vi "NanoBright Acquisition self-aligning source code.vi"(1 "Acquisition\nTime (s)":u32=10, 2 "Number \nof files":i32=5 min=1 max=99 step=1, 3 "Acquisition Rate (Hz)":dbl=1000.0 caption="Acquisition\nRate (Hz)") -> ()   [LabVIEW 2014]
uses:
  C:/Program Files (x86)/National Instruments/LabVIEW 2014/vi.lib/ULx/ULx_LV.dll
  Program Files (x86)/National Instruments/LabVIEW 2014/vi.lib/ULx/ULx_LV.dll
  <vilib>/Utility/error.llb/DialogType.ctl
  <vilib>/Analysis/baseanly.llb/Mean (DBL).vi
  <vilib>/ULx/Create Channel.llb/ULx Create Channel (CI-Count Edges).vi
  <vilib>/ULx/Timing.llb/ULx Timing (Sample Clock).vi
  <vilib>/ULx/Read.llb/ULx Read (Counter 1D U32 1Chan NSamp).vi
  <vilib>/Utility/file.llb/Read From Spreadsheet File (DBL).vi
  <vilib>/Analysis/NI_AALBase.lvlib
panel:
  in  "Instrument Key":string="COM3"
  in  "Align after # of loops":dbl=2.0
  in  "Period of measurement (min)":u32=1
  out "concatenated string":string="20_30"
  out "Buffer":dbl=100.0
  out "Samples/loop":i32=10
  in  "File Prefix":string="testa"
  out "Current File":i32=1 format="%1.0f"
  out "Channel 1":dbl=nan format="%#_3g"
  out "Signal":u32[][](graph)
  in  "Clock Source":i32(ring) items=["OnboardClock", "ExternalClock", "NoClock"]
  in  "Count Direction":i32(ring) items=["CountUp", "CountDown"]
  in  "Edge":i32(ring) items=["Rising", "Falling"]
  in  "Counter(s)":refnum<k21>="Dev0/Ci0"
  in  "Initial Count":u32
  in  "stop":bool
  # "Signal Averages"
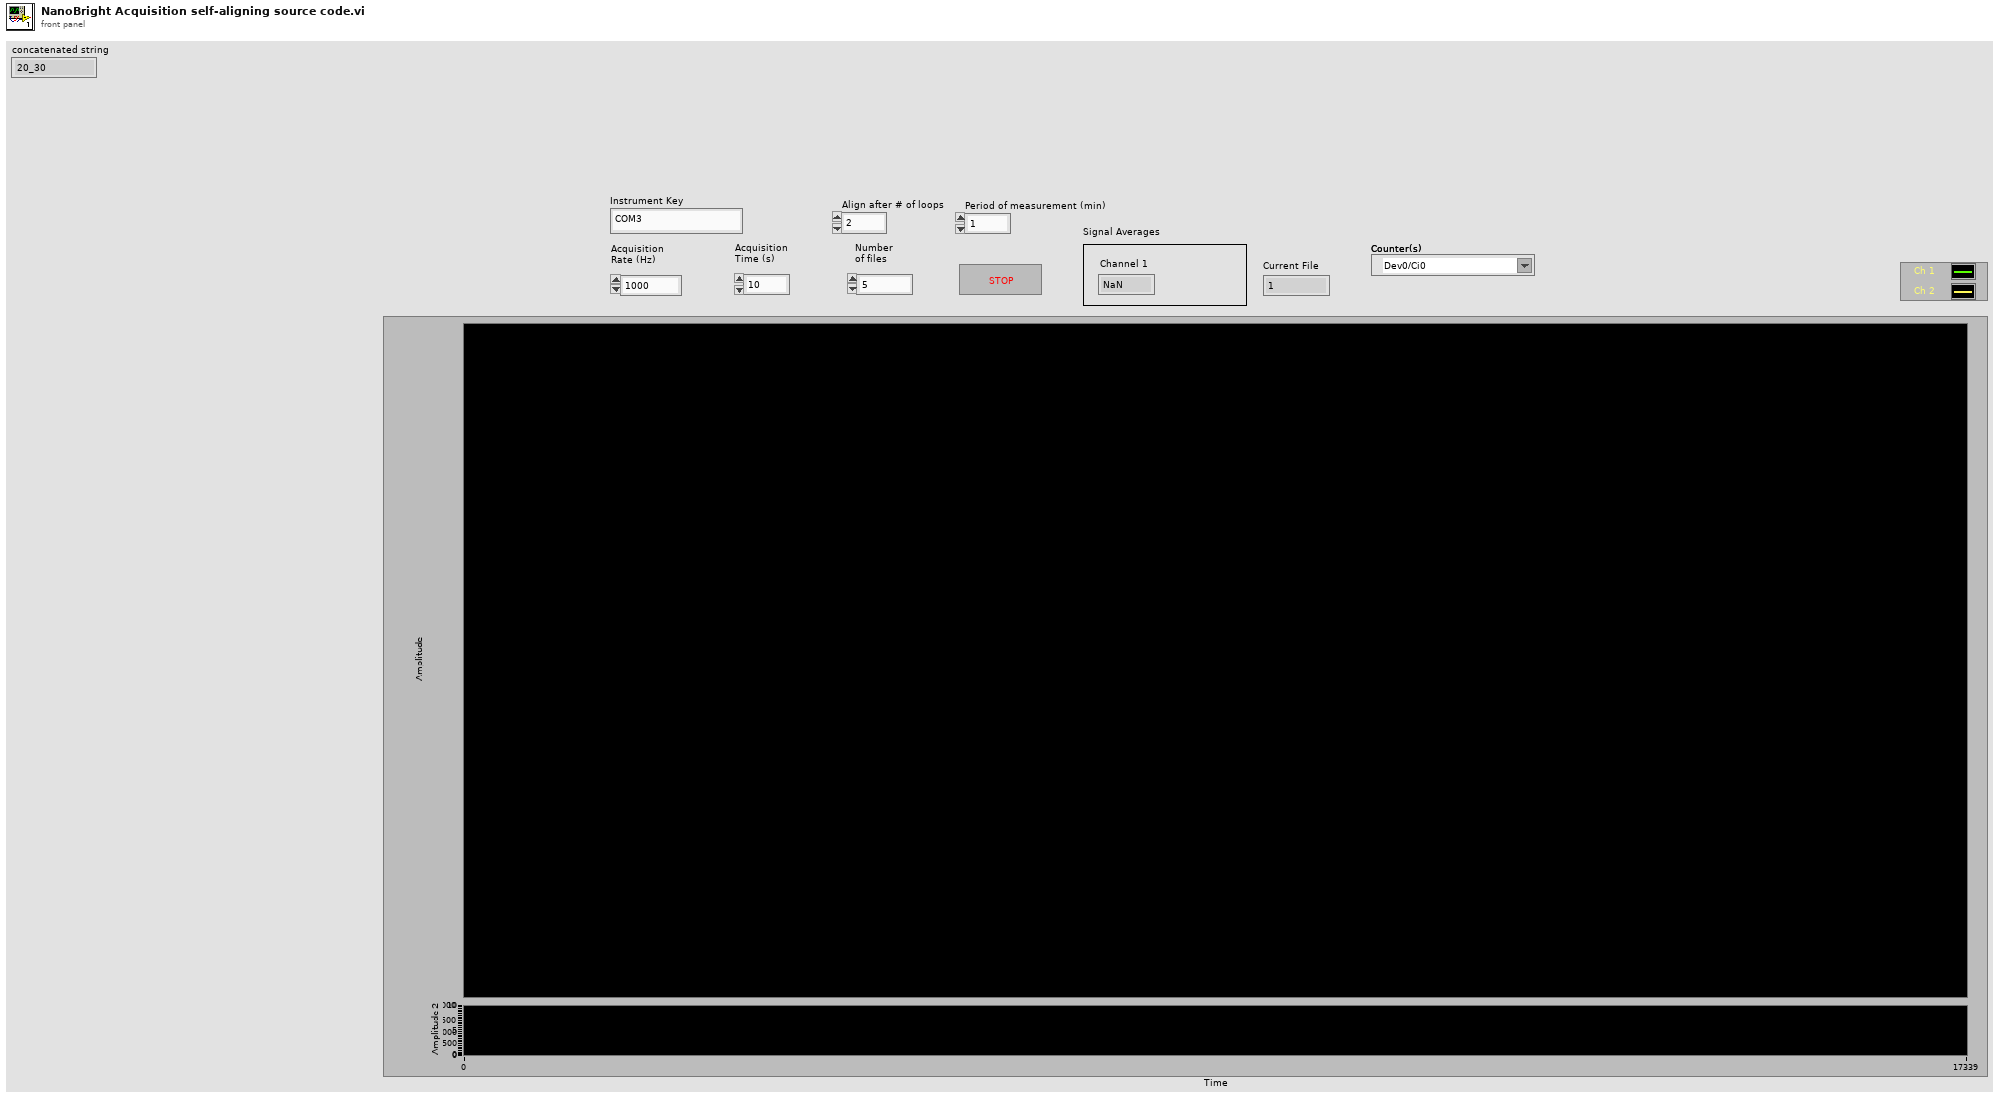
[diagram p1: front panel]
types:
  T1 = enum16{"open", "replace", "create", "open or create", "replace or create", "replace or create with confirmation"}
  T2 = typedef "DialogType.ctl" = u16
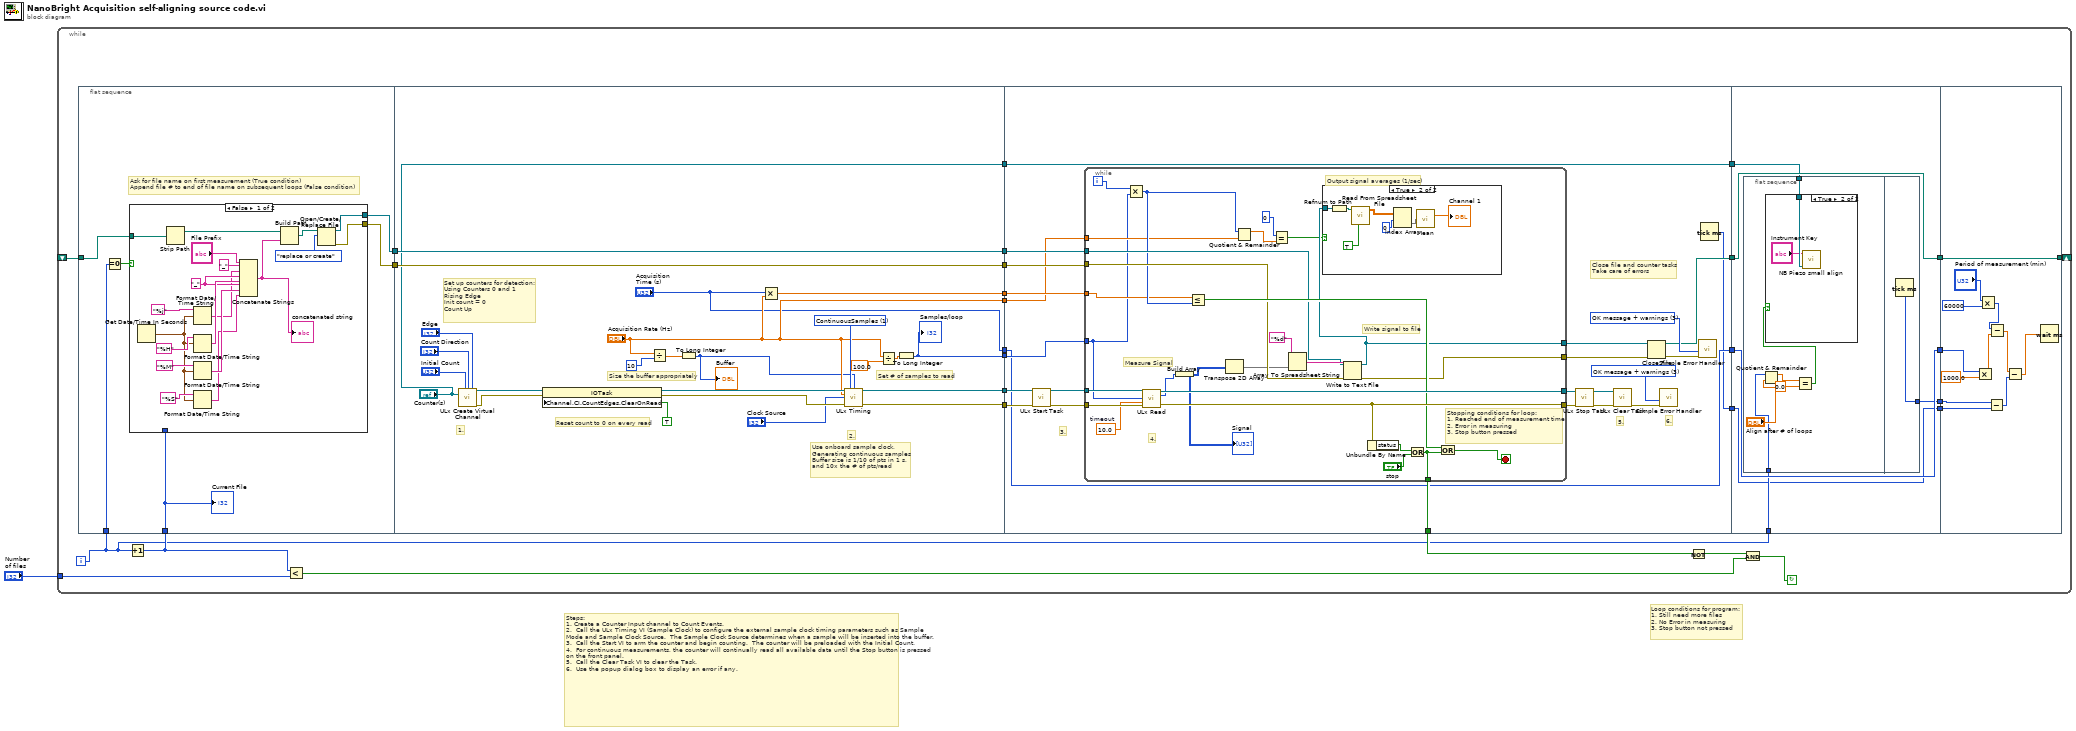
[diagram p0: block diagram]
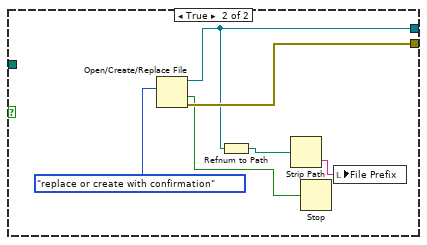
[diagram p2: hidden frame]
diagram:
  # "Loop conditions for program:\n1. Still need more files\n2. No Error in measuring\n3. Stop button not pressed"
  # "Steps: \n1. Create a Counter Input channel to Count Events.\n2.  Call the ULx Timing VI (Sample Clock) to configure the external sample clock timing parameters such as Sample Mode and Sample Clock Source.  The Sample Clock Source determines when a sample will be inserted into the buffer.\n3.  Call the Start VI to arm the counter and begin counting.  The counter will be preloaded with the Initial Count.\n4.  For continuous measurements, the counter will continually read all available data until the Stop button is pressed on the front panel.\n5.  Call the Clear Task VI to clear the Task.\n6.  Use the popup dialog box to display an error if any."
  n1 = while {
    tunnel: "Number \nof files" -> [w21]
    shift-right: [w16] -> _
    shift-left: _ -> [w17]
    i -> [w7]
    stop <- w20 continue-if-true
    n2 = flat-sequence {
      tunnel: [w32] -> w29
      tunnel: [w31] -> w28
      tunnel: w22 -> [w33]
      tunnel: w17 -> [w30]
      tunnel: w7 -> [w34]
      tunnel: [w84] -> w27
      tunnel: [w83] -> w26
      tunnel: [w74] -> w25
      tunnel: [w72] -> w24
      tunnel: [w73] -> w23
      tunnel: w29 -> [w84]
      tunnel: w28 -> [w83]
      tunnel: ["Acquisition Rate (Hz)"] -> w14
      tunnel: [w64] -> w13
      tunnel: ["Acquisition\nTime (s)"] -> w12
      tunnel: ["Counter(s)"] -> w5
      tunnel: w27 -> [w104]
      tunnel: w26 -> [w98]
      tunnel: w25 -> [w94]
      tunnel: w24 -> [w93]
      tunnel: w23 -> [w92]
      tunnel: [w91] -> w19
      tunnel: w14 -> [w89]
      tunnel: w13 -> [w88]
      tunnel: [w90] -> w11
      tunnel: w12 -> [w87]
      tunnel: [w87] -> w9
      tunnel: [w86] -> w6
      tunnel: w5 -> [w86]
      tunnel: [w85] -> w3
      tunnel: w11 -> [w148]
      tunnel: [w148] -> w10
      tunnel: w9 -> [w147]
      tunnel: [w147] -> w8
      tunnel: w7 -> [w146]
      tunnel: w6 -> [w145]
      tunnel: [w144] -> w4
      tunnel: w3 -> [w144]
      tunnel: [w143] -> w2
      tunnel: [w169] -> w16
      tunnel: w10 -> [w169]
      tunnel: w8 -> [w163]
      tunnel: w4 -> [w161]
      tunnel: w2 -> [w162]
      frame #0 {
        # "Ask for file name on first measurement (True condition)\nAppend file # to end of file name on subsequent loops (False condition)"
        n3 = Equal To 0?(x=w34) -> (x = 0?=w35:bool)
        n4 = case shown="False" w35 {
          tunnel: [w50 w60] -> w31
          tunnel: [w49 w58] -> w32
          tunnel: w30 -> [w54 _]
          tunnel: w33 -> [_ _]
          frame False {
            w40 = "_" ("string")
            n5 = Get Date/Time In Seconds() -> (seconds since 1Jan1904=w37:timestamp)
            n6 = Strip Path(path=w54) -> (stripped path=w53:path)  [unwired: 1 out]
            n7 = Format Date/Time String(time format string (%c)="%j", seconds (now)=w37) -> (date/time string=w39:string)  [unwired: 1 in]
            n8 = Format Date/Time String(time format string (%c)="%H", seconds (now)=w37) -> (date/time string=w41:string)  [unwired: 1 in]
            n9 = Format Date/Time String(time format string (%c)="%M", seconds (now)=w37) -> (date/time string=w42:string)  [unwired: 1 in]
            n10 = Format Date/Time String(time format string (%c)="%S", seconds (now)=w37) -> (date/time string=w36:string)  [unwired: 1 in]
            n11 = Concatenate Strings("File Prefix", "_" ("string"), w39, w40, w41, w40, w42, w36) -> (w44:string)
            "concatenated string" <- w44
            n12 = Build Path(base path=w53, name or relative path=w44) -> (appended path=w52:path)
            n13 = Open/Create/Replace File(file path (use dialog)=w52, operation (0:open)=T1."replace or create") -> (refnum out=w49:refnum<file>, error out=w50:errorcluster)  [unwired: 4 in, 1 out]
          }
          frame True {
            n14 = Open/Create/Replace File(operation (0:open)=T1."replace or create with confirmation") -> (refnum out=w58:refnum<file>, cancelled=w55:bool, error out=w60:errorcluster)  [unwired: 5 in]
            n15 = Refnum to Path(1:w58) -> (0:w57:path)
            n16 = Strip Path(path=w57) -> (name=w56:string)  [unwired: 1 out]
            n17 = Stop(stop? (T)=w55) -> ()
            n18 = local write "File Prefix"(w56) -> ()
          }
        }
        "Current File" <- w33
      }
      frame #1 {
        w75 = 1 items=["FiniteSamples", "ContinuousSamples"] ("sample mode")
        # "Use onboard sample clock,\nGenerating continuous samples\nBuffer size is 1/10 of pts in 1 s, \nand 10x the # of pts/read"
        # "Reset count to 0 on every read"
        # "Set up counters for detection:\nUsing Counters 0 and 1\nRising Edge\nInit count = 0\nCount Up"
        # "Set # of samples to read"
        # "Size the buffer appropriately"
        # "2."
        # "1."
        n19 = call-poly <vilib>:"ULx Create Virtual Channel.vi"("initial count"="Initial Count", "count direction"="Count Direction", "edge"="Edge", "counters"="Counter(s)") -> ("task out"=w71:refnum<k24>, "error out"=w70:errorcluster)  [unwired: 10 in]
        n20 = property class="IOTask"(reference=w71, error in=w70, "Channel.CI.CountEdges.ClearOnRead"=TRUE) -> (reference out=w81:refnum<k24>, error out=w82:errorcluster)
        n21 = Divide(x="Acquisition Rate (Hz)", y=10 ("samples per channel")) -> (x/y=w68:dbl)
        n22 = To Long Integer(number=w68) -> (32bit integer=w63:i32)
        "Buffer" <- w63
        n23 = Multiply(x="Acquisition\nTime (s)", y="Acquisition Rate (Hz)") -> (x*y=w74:dbl)
        n24 = call-poly <vilib>:"ULx Timing.vi"("task in"=w81, "sample mode"=w75, "samples per channel"=w63, "rate"="Acquisition Rate (Hz)", "clock source"="Clock Source", "error in"=w82) -> ("task out"=w73:refnum<k24>, "error out"=w72:errorcluster)  [unwired: 8 in]
        n25 = Divide(x="Acquisition Rate (Hz)", y=100.0) -> (x/y=w65:dbl)
        n26 = To Long Integer(number=w65) -> (32bit integer=w64:i32)
        "Samples/loop" <- w64
      }
      frame #2 {
        w95 = T2 3 items=["no dialog", "OK message", "continue or stop message", "OK message + warnings", "continue/stop + warnings"] ("type of dialog (OK msg:1)")
        w105 = T2 3 items=["no dialog", "OK message", "continue or stop message", "OK message + warnings", "continue/stop + warnings"] ("type of dialog (OK msg:1)")
        # "Close file and counter tasks\nTake care of errors"
        # "6."
        # "5."
        # "3."
        n27 = call <vilib>:"ULx Start Task.vi"("task in"=w92, "error in"=w93) -> ("task out"=w106:refnum<k24>, "error out"=w108:errorcluster)  [unwired: 12 in]
        n28 = while {
          tunnel: w108 -> [w135]
          tunnel: [w129] -> w101
          tunnel: w106 -> [w132]
          tunnel: [w130] -> w102
          tunnel: w104 -> [w123]
          tunnel: [w122] -> w103
          tunnel: w98 -> [w125]
          tunnel: [w124] -> w97
          tunnel: w94 -> [w117]
          tunnel: [w115] -> w91
          tunnel: w89 -> [w114]
          tunnel: w88 -> [w113]
          i -> [w112]
          stop <- w116 stop-if-true
          w131 = 10.0  # timeout
          # "Output signal averages (1/sec)"
          # "Stopping conditions for loop:\n1. Reached end of measurement time\n2. Error in measuring\n3. Stop button pressed"
          # "Measure Signal"
          # "Write signal to file"
          # "4."
          n29 = Multiply(x=w112, y=w113) -> (x*y=w121:i32)
          n30 = call-poly <vilib>:"ULx Read.vi"("task in"=w132, "number of samples per channel"=w113, "timeout"=w131, "error in"=w135) -> ("task out"=w130:refnum<k24>, "data"=w111:u32[], "error out"=w129:errorcluster)  [unwired: 9 in]
          n31 = Build Array(w111) -> (w110:u32[][])
          "Signal" <- w110
          n32 = Less Or Equal?(x=w117, y=w121) -> (x <= y?=w126:bool)
          n33 = Transpose 2D Array(2D array=w110) -> (transposed array=w109:u32[][])
          n34 = Quotient & Remainder(x=w121, y=w114) -> (x-y*floor(x/y)=w120:dbl)  [unwired: 1 out]
          n35 = Equal?(x=0, y=w120) -> (x = y?=w118:bool)
          n36 = Array To Spreadsheet String(array=w109, 3:"%d" ("format string")) -> (spreadsheet string=w128:string)  [unwired: 1 in]
          n37 = Write to Text File(file (use dialog)=w123, text=w128, error in=w125) -> (refnum out=w122:refnum<file>, error out=w124:errorcluster)  [unwired: 1 in, 1 out]
          n38 = case shown="True" w118 {
            tunnel: w122 -> [_ w136]
            frame False {
            }
            frame True {
              n39 = Refnum to Path(1:w136) -> (0:w140:path)
              n40 = call-poly <vilib>:"Read From Spreadsheet File.vi"("transpose (no:F)"=TRUE, "file path (dialog if empty)"=w140) -> ("all rows"=w139:dbl[][])  [unwired: 5 in, 4 out]
              n41 = Index Array(array=w139, index (row)=0) -> (element=w141:dbl[])  [unwired: 1 in]
              n42 = call-poly <vilib>:"Mean.vi"("X"=w141) -> ("mean"=→"Channel 1":dbl)  [unwired: 1 out]
            }
          }
          n43 = Unbundle By Name(w129) -> ("status"=w133:bool)
          n44 = Or(x=w133, y="stop") -> (x .or. y?=w115:bool)
          n45 = Or(x=w126, y=w115) -> (x .or. y?=w116:bool)
        }
        n46 = call <vilib>:"ULx Stop Task.vi"("error in"=w101, "task in"=w102) -> ("error out"=w99:errorcluster, "task out"=w100:refnum<k24>)  [unwired: 8 in]
        n47 = call <vilib>:"ULx Clear Task.vi"("task in"=w100, "error in"=w99) -> ("error out"=w107:errorcluster)  [unwired: 13 in]
        n48 = Close File(refnum=w103, error in=w97) -> (path=w90:path, error out=w96:errorcluster)
        n49 = call <vilib>:"Simple Error Handler.vi"("type of dialog (OK msg:1)"=w105, "error in (no error)"=w107) -> ()  [unwired: 3 in, 5 out]
        n50 = call <vilib>:"Simple Error Handler.vi"("type of dialog (OK msg:1)"=w95, "error in (no error)"=w96) -> ()  [unwired: 3 in, 5 out]
        n51 = Tick Count (ms)() -> (millisecond timer value=w85:u32)
      }
      frame #3 {
        n52 = flat-sequence {
          tunnel: w146 -> [w150]
          tunnel: w145 -> [w149]
          tunnel: [w157] -> w143
          frame #0 {
            n53 = Quotient & Remainder(x=w150, y="Align after # of loops") -> (x-y*floor(x/y)=w154:dbl)  [unwired: 1 out]
            n54 = Equal?(x=w154, y=0.0) -> (x = y?=w152:bool)
            n55 = case shown="True" w152 {
              tunnel: w149 -> [_ w156]
              frame False {
              }
              frame True {
                n56 = call "NB Piezo small align.vi"("Counter(s)"=w156, "Instrument Key"="Instrument Key") -> ()  [unwired: 2 in]
              }
            }
          }
          frame #1 {
            n57 = Tick Count (ms)() -> (millisecond timer value=w157:u32)
          }
        }
      }
      frame #4 {
        n58 = Multiply(x=w163, y=1000.0) -> (x*y=w164:dbl)
        n59 = Multiply(x="Period of measurement (min)", y=u32 60000) -> (x*y=w166:u32)
        n60 = Subtract(x=w162, y=w161) -> (x-y=w159:u32)
        n61 = Subtract(x=w166, y=w164) -> (x-y=w160:dbl)
        n62 = Subtract(x=w160, y=w159) -> (x-y=w158:dbl)
        n63 = Wait (ms)(milliseconds to wait=w158) -> ()  [unwired: 1 out]
      }
    }
    n64 = Increment(x=w7) -> (x+1=w22:i32)
    n65 = Less?(x=w22, y=w21) -> (x < y?=w15:bool)
    n66 = Not(x=w19) -> (.not. x?=w18:bool)
    n67 = And(x=w18, y=w15) -> (x .and. y?=w20:bool)
  }
